vi "Parse Master USB Packet.vi"() -> ()   [LabVIEW 2026]
uses:
  Real Wind Sample.ctl
panel:
  out "Packet Valid?":bool
  in  "Wind Sample":T1
  in  "Raw Master Packet":string
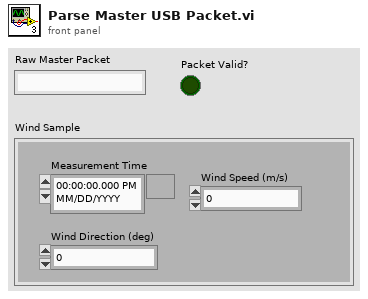
[diagram p1: front panel]
types:
  T1 = typedef "Real Wind Sample.ctl" = cluster{"Measurement Time":timestamp, "Wind Direction (deg)":dbl, "Wind Speed (m/s)":dbl}
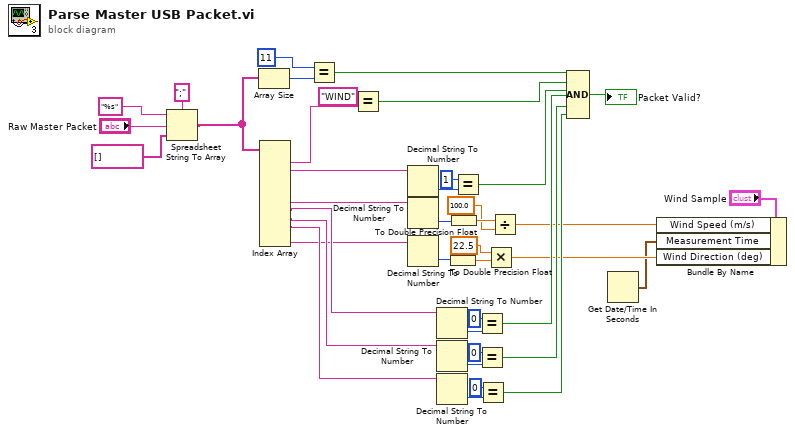
[diagram p0: block diagram]
diagram:
  n1 = Spreadsheet String To Array(delimiter (Tab)=";", format string="%s", spreadsheet string="Raw Master Packet", array type (2D Dbl)=string[] []) -> (array=w36:string[])
  n2 = Array Size(array=w36) -> (size(s)=w35:i32)
  n3 = Index Array(array=w36) -> (element #1=w33:string, element #2=w29:string, element #6=w28:string, element #7=w27:string, element #8=w31:string, element #9=w30:string, element #11=w26:string)  [unwired: 11 in, 4 out]
  n4 = Equal?(x=11, y=w35) -> (x = y?=w11:bool)
  n5 = Equal?(x="WIND", y=w33) -> (x = y?=w10:bool)
  n6 = Decimal String To Number(string=w29) -> (number=w25:i32)  [unwired: 2 in, 1 out]
  n7 = Decimal String To Number(string=w28) -> (number=w23:i32)  [unwired: 2 in, 1 out]
  n8 = Decimal String To Number(string=w26) -> (number=w20:i32)  [unwired: 2 in, 1 out]
  n9 = Decimal String To Number(string=w27) -> (number=w17:i32)  [unwired: 2 in, 1 out]
  n10 = Decimal String To Number(string=w31) -> (number=w16:i32)  [unwired: 2 in, 1 out]
  n11 = Decimal String To Number(string=w30) -> (number=w15:i32)  [unwired: 2 in, 1 out]
  n12 = To Double Precision Float(number=w20) -> (double precision float=w19:dbl)
  n13 = To Double Precision Float(number=w23) -> (double precision float=w22:dbl)
  n14 = Equal?(x=1, y=w25) -> (x = y?=w9:bool)
  n15 = Equal?(x=0, y=w17) -> (x = y?=w8:bool)
  n16 = Equal?(x=0, y=w16) -> (x = y?=w7:bool)
  n17 = Equal?(x=0, y=w15) -> (x = y?=w6:bool)
  n18 = Multiply(x=22.5, y=w19) -> (x*y=w3:dbl)
  n19 = Divide(x=w22, y=100.0) -> (x/y=w2:dbl)
  n20 = Compound Arithmetic op=AND(w11, w10, w9, w8, w7, w6) -> (→"Packet Valid?":bool)
  n21 = Get Date/Time In Seconds() -> (seconds since 1Jan1904=w1:timestamp)
  n22 = Bundle By Name(cluster="Wind Sample", "Wind Speed (m/s)"=w2, "Measurement Time"=w1, "Wind Direction (deg)"=w3) -> ()  [unwired: 1 out]
